vi "ReceiveMIMICCommand.vi"(0 "error in":errorcluster, 1 "Desired_Length":u32, 2 "CheckSum?":bool=TRUE, 3 "Timeout":u32=5000) -> (4 "Receive_buffer":u8[](array[numeric]), 5 "error out":errorcluster, 6 "Success?":bool, 7 "BytesToRead":u32, 8 "Read Time":u32)   [LabVIEW 2014]
panel:
  out "STRT_TIME":u32
  # "NOTE.- Desired_Length variable controls how many bytes are going to be read\nfrom the RS-232 comport. If this variable is set to ZERO, the number of bytes to read\nwill be obtained from the first byte in the response (MIMIC Protocol)"
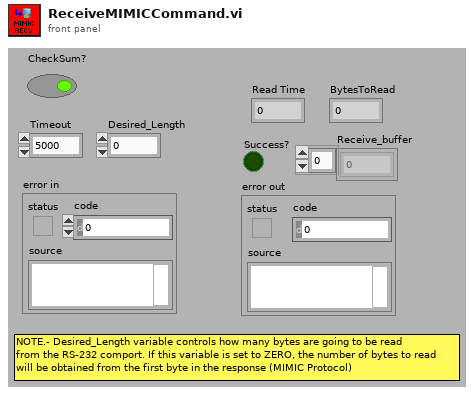
[diagram p1: front panel]
types:
  T1 = enum16{"OpenPort", "Initial Serial Port", "Write", "ByteRead", "Read", "ClearBuff", "Close"}
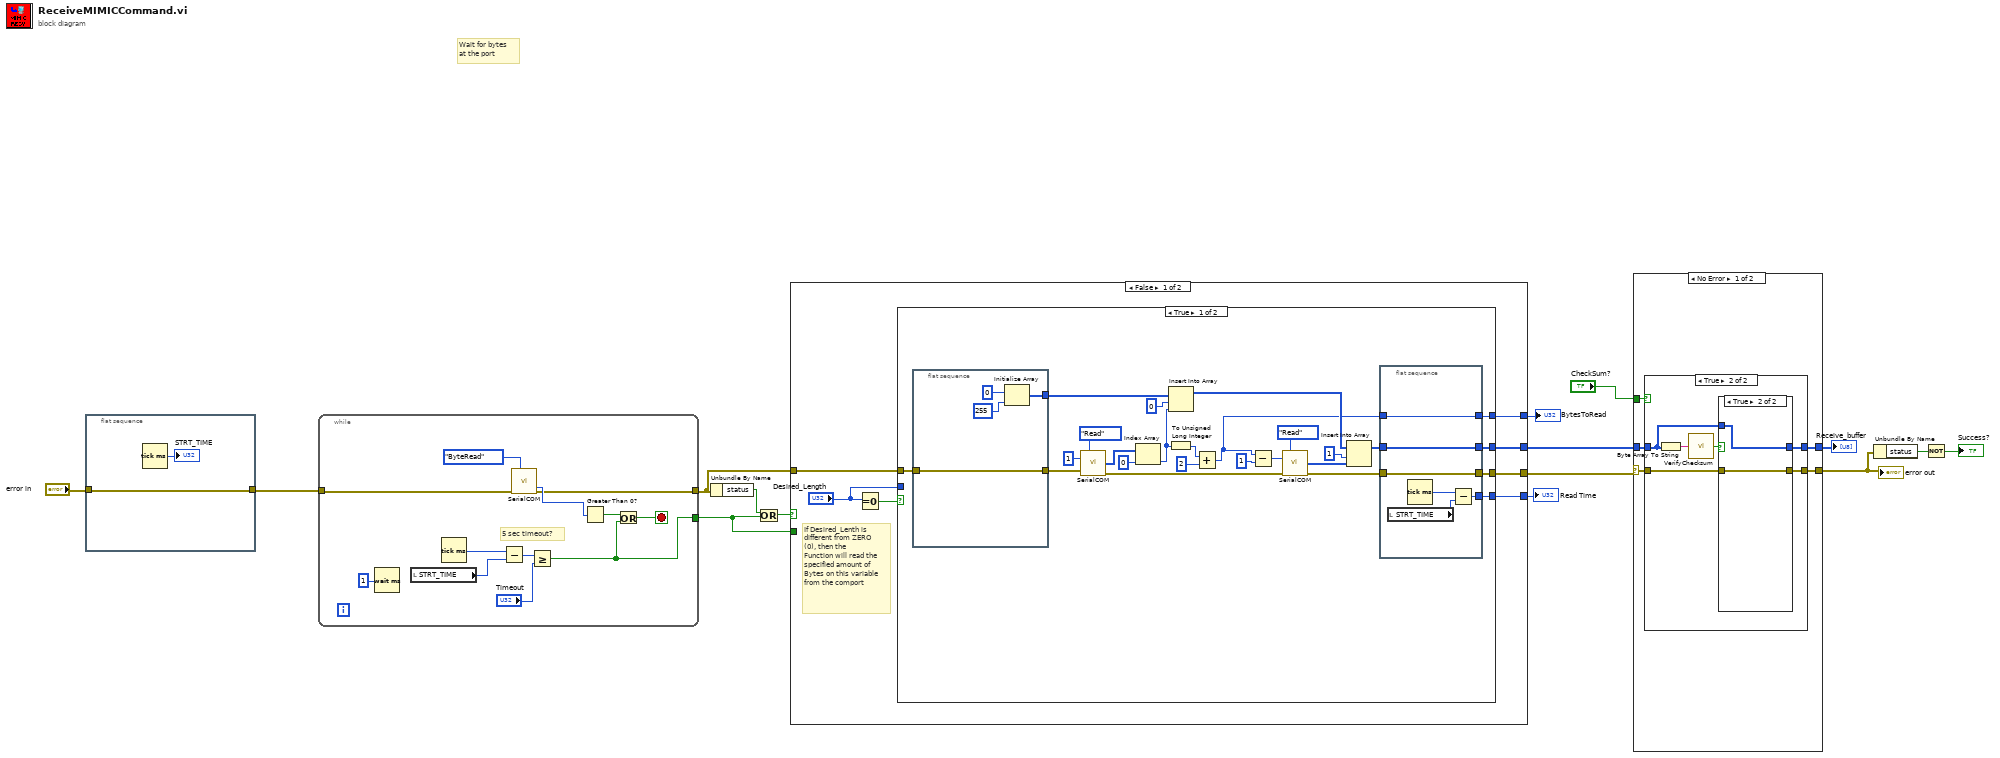
[diagram p0: block diagram]
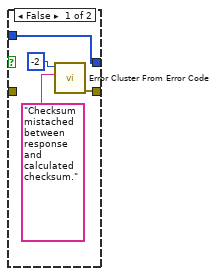
[diagram p3: hidden frame]
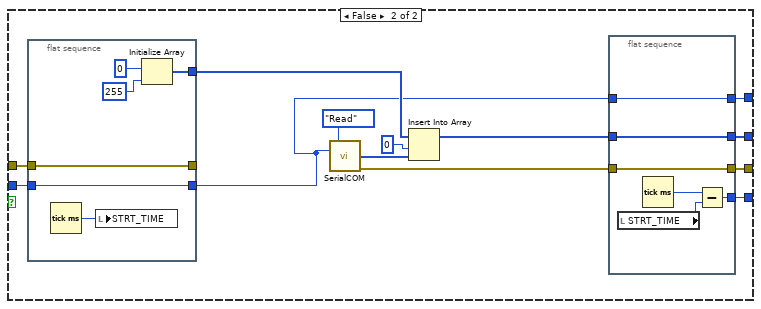
[diagram p5: hidden frame]
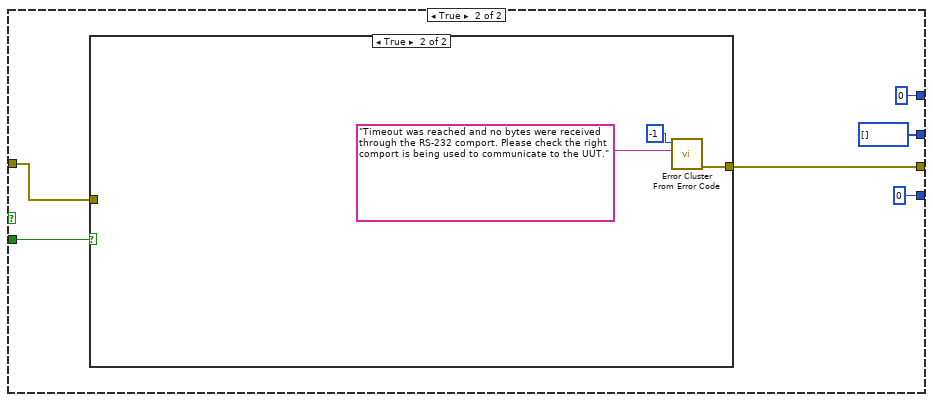
[diagram p6: hidden frame]
diagram:
  # "Wait for bytes\nat the port"
  n1 = flat-sequence {
    tunnel: "error in" -> [w16]
    tunnel: [w16] -> w14
    frame #0 {
      n2 = Tick Count (ms)() -> (millisecond timer value=→"STRT_TIME":u32)
    }
  }
  n3 = while {
    tunnel: w14 -> [w20]
    tunnel: [w19] -> w10
    tunnel: [w23] -> w11
    stop <- w29 stop-if-true
    # "5 sec timeout?"
    n4 = Wait (ms)(milliseconds to wait=u32 1 ("millisecond multiple")) -> ()  [unwired: 1 out]
    n5 = local read "STRT_TIME"() -> (w24:u32)
    n6 = Tick Count (ms)() -> (millisecond timer value=w26:u32)
    n7 = Subtract(x=w26, y=w24) -> (x-y=w25:u32)
    n8 = call "SerialCOM.vi"("Function"=T1."ByteRead", "error in (no error)"=w20) -> ("Bytes at Port"=w21:u32, "error out"=w19:errorcluster)  [unwired: 8 in, 4 out]
    n9 = Greater Or Equal?(x=w25, y="Timeout") -> (x >= y?=w23:bool)
    n10 = Greater Than 0?(x=w21) -> (x > 0?=w27:bool)
    n11 = Or(x=w27, y=w23) -> (x .or. y?=w29:bool)
  }
  n12 = Unbundle By Name(w10) -> ("status"=w12:bool)
  n13 = Or(x=w12, y=w11) -> (x .or. y?=w13:bool)
  n14 = case shown="False" w13 {
    tunnel: w11 -> [_ w102]
    tunnel: w10 -> [w36 w101]
    tunnel: [w35 u32 0] -> w9
    tunnel: [w33 u8[] []] -> w6
    tunnel: [w34 w100] -> w7
    tunnel: [w31 u32 0 ("Desired_Length")] -> w8
    frame False {
      # "If Desired_Lenth is different from ZERO (0), then the Function will read the specified amount of Bytes on this variable from the comport"
      n15 = Equal To 0?(x="Desired_Length") -> (x = 0?=w32:bool)
      n16 = case shown="True" w32 {
        tunnel: w36 -> [w61 w84]
        tunnel: [w41 w78] -> w35
        tunnel: [w40 w77] -> w34
        tunnel: [w39 w76] -> w33
        tunnel: [w37 w72] -> w31
        tunnel: "Desired_Length" -> [_ w74]
        frame True {
          n17 = flat-sequence {
            tunnel: [w69] -> w60
            tunnel: w61 -> [w69]
            tunnel: [w68] -> w49
            frame #0 {
              n18 = Initialize Array(u8 0 ("element"), 255 ("dimension size")) -> (w68:u8[])
            }
          }
          n19 = call "SerialCOM.vi"("Function"=T1."Read", "byte count"=u32 1, "error in (no error)"=w60) -> ("array Out"=w54:u8[], "error out"=w50:errorcluster)  [unwired: 7 in, 4 out]
          n20 = Index Array(array=w54, index=0) -> (element=w47:u8)
          n21 = Insert Into Array(array=w49, index=0, new element=w47) -> (w46:u8[])
          n22 = To Unsigned Long Integer(number=w47) -> (unsigned 32bit integer=w55:u32)
          n23 = Add(x=w55, y=u32 2) -> (x+y=w38:u32)
          n24 = Subtract(x=w38, y=u32 1) -> (x-y=w52:u32)
          n25 = call "SerialCOM.vi"("Function"=T1."Read", "byte count"=w52, "error in (no error)"=w50) -> ("array Out"=w44:u8[], "error out"=w43:errorcluster)  [unwired: 7 in, 4 out]
          n26 = Insert Into Array(array=w46, index=1, new element=w44) -> (w42:u8[])
          n27 = flat-sequence {
            tunnel: [w65] -> w40
            tunnel: w43 -> [w65]
            tunnel: [w64] -> w39
            tunnel: w42 -> [w64]
            tunnel: [w63] -> w41
            tunnel: w38 -> [w62]
            tunnel: [w62] -> w37
            frame #0 {
              n28 = local read "STRT_TIME"() -> (w66:u32)
              n29 = Tick Count (ms)() -> (millisecond timer value=w67:u32)
              n30 = Subtract(x=w67, y=w66) -> (x-y=w63:u32)
            }
          }
        }
        frame False {
          n31 = flat-sequence {
            tunnel: [w93] -> _
            tunnel: w84 -> [w93]
            tunnel: [w92] -> w75
            tunnel: w74 -> [w91]
            tunnel: [w91] -> w73
            frame #0 {
              n32 = Tick Count (ms)() -> (millisecond timer value=w96:u32)
              n33 = local write "STRT_TIME"(w96) -> ()
              n34 = Initialize Array(u8 0 ("element"), 255 ("dimension size")) -> (w92:u8[])
            }
          }
          n35 = call "SerialCOM.vi"("Function"=T1."Read", "byte count"=w73) -> ("array Out"=w81:u8[], "error out"=w80:errorcluster)  [unwired: 8 in, 4 out]
          n36 = Insert Into Array(array=w75, index=0, new element=w81) -> (w79:u8[])
          n37 = flat-sequence {
            tunnel: [w88] -> w77
            tunnel: w80 -> [w88]
            tunnel: [w87] -> w76
            tunnel: w79 -> [w87]
            tunnel: [w86] -> w78
            tunnel: [w85] -> w72
            tunnel: w73 -> [w85]
            frame #0 {
              n38 = local read "STRT_TIME"() -> (w89:u32)
              n39 = Tick Count (ms)() -> (millisecond timer value=w90:u32)
              n40 = Subtract(x=w90, y=w89) -> (x-y=w86:u32)
            }
          }
        }
      }
    }
    frame True {
      n41 = case shown="True" w102 {
        tunnel: [w103 w104] -> w100
        tunnel: w101 -> [w103 _]
        frame False {
        }
        frame True {
          n42 = call <vilib>:"Error Cluster From Error Code.vi"("error message (\"\")"="Timeout was reached and no bytes were received through the RS-232 comport. Please check the right comport is being used to communicate to the UUT." ("error message (\"\")"), "error code (0)"=-1) -> ("error out"=w104:errorcluster)  [unwired: 7 in]
        }
      }
    }
  }
  "Read Time" <- w9
  "BytesToRead" <- w8
  n43 = case shown="No Error" w7 {
    selector: w7 -> [w107 w127]
    tunnel: [w108 w127] -> w3
    tunnel: [w109 w126] -> w5
    tunnel: w6 -> [w110 w126]
    tunnel: "CheckSum?" -> [w111 _]
    frame No Error {
      n44 = case shown="True" w111 {
        tunnel: w110 -> [w113 w115]
        tunnel: [w113 w114] -> w109
        tunnel: [w112 w116] -> w108
        tunnel: w107 -> [w112 w117]
        frame False {
        }
        frame True {
          n45 = Byte Array To String(unsigned byte array=w115) -> (string=w119:string)
          n46 = call "VerifyChecksum.vi"("HEX String to Verify CheckSum"=w119) -> ("Success?"=w118:bool)
          n47 = case shown="True" w118 {
            tunnel: [w122 w125] -> w116
            tunnel: w117 -> [_ w125]
            tunnel: w115 -> [w123 w124]
            tunnel: [w123 w124] -> w114
            frame False {
              n48 = call <vilib>:"Error Cluster From Error Code.vi"("error message (\"\")"="Checksum mistached between response and calculated checksum." ("error message (\"\")"), "error code (0)"=-2) -> ("error out"=w122:errorcluster)  [unwired: 7 in]
            }
            frame True {
            }
          }
        }
      }
    }
    frame Error {
    }
  }
  "error out" <- w3
  "Receive_buffer" <- w5
  n49 = Unbundle By Name(w3) -> ("status"=w2:bool)
  n50 = Not(x=w2) -> (.not. x?=→"Success?":bool)
